vi "prototype-01.vi"() -> ()   [LabVIEW 2026]
uses:
  <vilib>/Instr/_visa.llb/VISA Configure Serial Port (Instr).vi
panel:
  in  "VISA resource name":refnum<visa-resource-name>
  in  "stop":bool
  in  "Current":dbl(knob) scale=0.0..10.0
  in  "Voltage":dbl(knob) scale=0.0..250.0
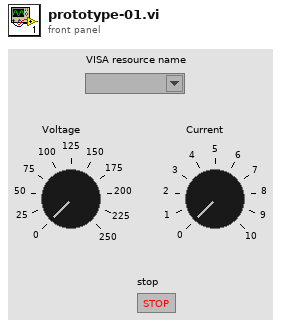
[diagram p1: front panel]
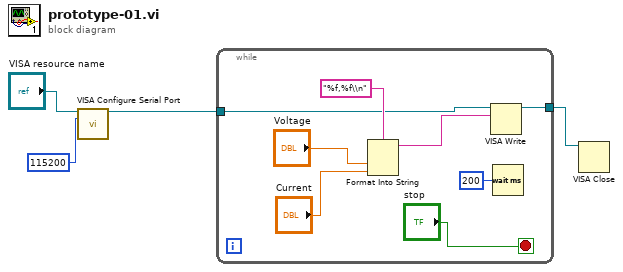
[diagram p0: block diagram]
diagram:
  n1 = call-poly "VISA Configure Serial Port"("VISA resource name"="VISA resource name", "baud rate (9600)"=u32 115200) -> ("VISA resource name out"=w2:refnum<visa-resource-name>)  [unwired: 12 in, 1 out]
  n2 = while {
    tunnel: w2 -> [w7]
    tunnel: [w6] -> w1
    stop <- "stop" stop-if-true
    n3 = Format Into String "Format Into String"(format string="%f,%f\\n", "Voltage", "Current") -> (resulting string=w8:string)  [unwired: 2 in, 1 out]
    n4 = VISA Write(VISA resource name=w7, write buffer=w8) -> (VISA resource name out=w6:refnum<visa-resource-name>)  [unwired: 1 in, 2 out]
    n5 = Wait (ms)(milliseconds to wait=u32 200) -> ()  [unwired: 1 out]
  }
  n6 = VISA Close(VISA resource name=w1) -> ()  [unwired: 1 in, 1 out]
